vi "testSendCmdStatus.vi"(8 "error in (no error)":errorcluster) -> (0 "error out":errorcluster)   [LabVIEW 2018]
doc: "Test the sendCmdStatus.vi."
uses:
  src/TcpServer/TcpServer.lvclass
  <vilib>/addons/_JKI Toolkits/Caraya/classes/Assert/Assert Equal Value_Variant.vi
  <vilib>/addons/_JKI Toolkits/Caraya/classes/Test/Test.lvclass
  <vilib>/addons/_JKI Toolkits/Caraya/classes/Assert/Assert.lvclass
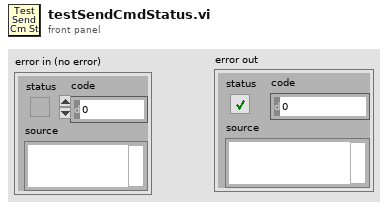
[diagram p1: front panel]
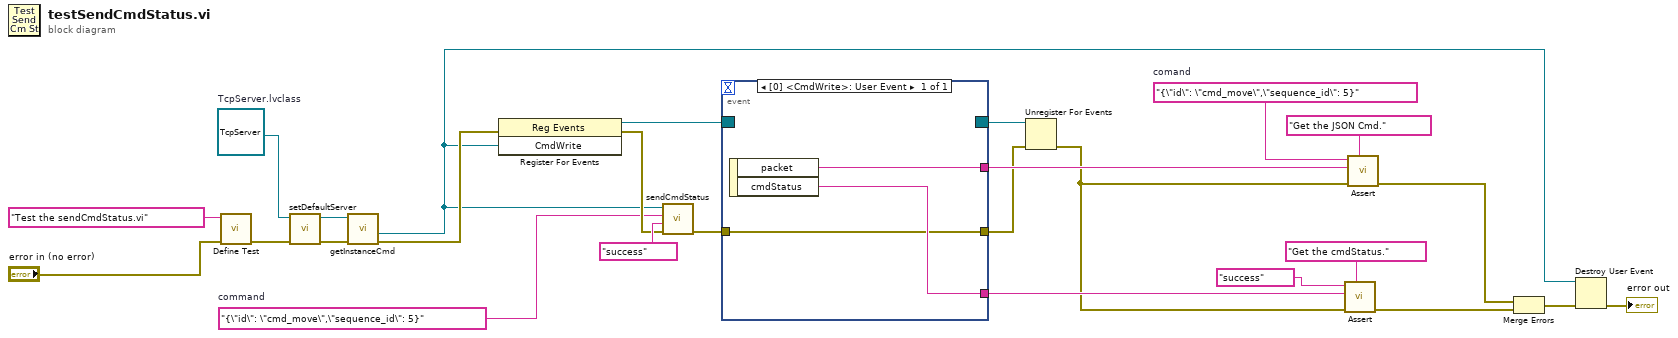
[diagram p0: block diagram]
diagram:
  w1 = "{\"id\": \"cmd_move\",\"sequence_id\": 5}"  # command
  w13 = "{\"id\": \"cmd_move\",\"sequence_id\": 5}"  # comand
  w23 = refnum<class "TcpServer.lvclass"> refnum  # TcpServer.lvclass
  n1 = call <vilib>:"Define Test.vi"("error in (no error)"="error in (no error)", "Label (VI Title)"="Test the sendCmdStatus.vi") -> ("error out"=w25:errorcluster)  [unwired: 9 in]
  n2 = call "setDefaultServer.vi"("error in (no error)"=w25, "TcpServer.lvclass"=w23) -> ("error out"=w3:errorcluster, "tcpServer out"=w4:refnum<class "TcpServer.lvclass">)  [unwired: 8 in]
  n3 = call "getInstanceCmd.vi"("error in (no error)"=w3, "tcpServer in"=w4) -> ("error out"=w5:errorcluster, "CmdWrite"=w2:refnum<user-event>)  [unwired: 6 in, 2 out]
  n4 = register-events(error in=w5, w2) -> (reference out=w21:refnum<event-registration>, error out=w20:errorcluster)  [unwired: 1 in]
  n5 = call "sendCmdStatus.vi"("error in (no error)"=w20, "cmdStatus"="success", "packet"=w1, "user event"=w2) -> ("error out"=w10:errorcluster)  [unwired: 7 in]
  n6 = event shown="[0] <CmdWrite>: User Event" {
    selector: w21 -> [_]
    dyn-events: [_] -> w9
    timeout: _ -> [_]
    tunnel: [w29] -> w17
    tunnel: [w28] -> w14
    tunnel: w10 -> [w27]
    tunnel: [w27] -> w8
    event User Event {
      n7 = event-data() -> ("packet"=w28:string, "cmdStatus"=w29:string)  [unwired: 1 in]
    }
  }
  n8 = Unregister For Events(event registration refnum=w9, error in=w8) -> (error out=w7:errorcluster)
  n9 = call-poly <vilib>:"Assert.vi"("Label"="Get the cmdStatus.", "error in (no error)"=w7, "Y"=w17, "X"="success" ("cmdStatus")) -> ("error out"=w12:errorcluster)  [unwired: 7 in]
  n10 = call-poly <vilib>:"Assert.vi"("Label"="Get the JSON Cmd.", "error in (no error)"=w7, "Y"=w14, "X"=w13) -> ("error out"=w11:errorcluster)  [unwired: 7 in]
  n11 = Merge Errors(w11, w12) -> (w19:errorcluster)
  n12 = Destroy User Event(user event=w2, error in=w19) -> (error out=→"error out":errorcluster)
